vi "Channels.Inline.Block Data Ref to Descriptor (Single).vi"(8 "error in (no error)":errorcluster, 11 "Block Data Ref":T3 {"Data Reference" format="%.0x"}) -> (0 "error out":errorcluster, 3 "Channel Block Descriptor":T1)   [LabVIEW 2016, in "VeriStand Data.lvlib"]
uses:
  VeriStand Data.lvlib
  <vilib>/NI Veristand/Custom Device API/Block Data Reference.ctl
  <vilib>/NI Veristand/Custom Device API/Data Reference.ctl
  Typedefs/Typedefs.Block Descriptor.Channel Block.ctl
  Typedefs/Typedefs.Block Descriptor.ctl
  Channels.Inline.Reference Error Handler.vi
  <vilib>/NI Veristand/Custom Device API/Global Data Refs.vi
  <vilib>/NI Veristand/Custom Device API/Custom Device API.lvlib
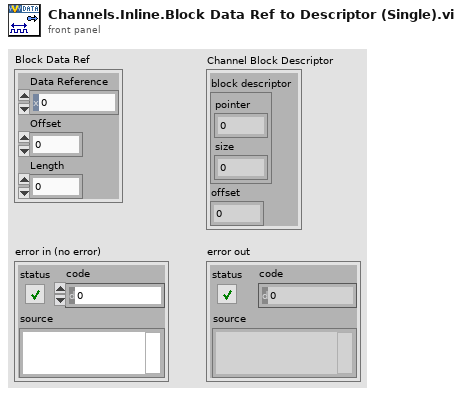
[diagram p1: front panel]
types:
  T1 = typedef "VeriStand Data.lvlib/Typedefs.Block Descriptor.Channel Block.ctl" = cluster{"block descriptor":T2, "offset":u64}
  T2 = typedef "VeriStand Data.lvlib/Typedefs.Block Descriptor.ctl" = cluster{"pointer":u64, "size":u64}
  T3 = typedef "Custom Device API.lvlib/Block Data Reference.ctl" = cluster{"Data Reference":T4, "Offset":u64, "Length":u64}
  T4 = typedef "Custom Device API.lvlib/Data Reference.ctl" = i32
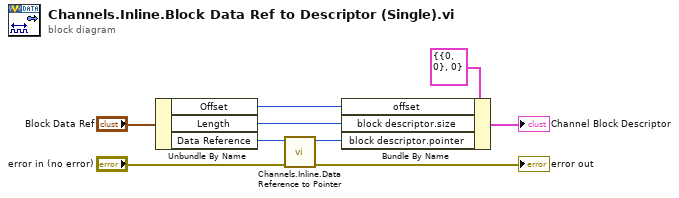
[diagram p0: block diagram]
diagram:
  n1 = Unbundle By Name("Block Data Ref") -> ("Offset"=w3:u64, "Length"=w6:u64, "Data Reference"=w9:T4)
  n2 = call "Channels.Inline.Data Reference to Pointer.vi"("error in (no error)"="error in (no error)", "Data Reference in"=w9) -> ("error out"=→"error out":errorcluster, "Channel Pointer"=w7:u64)  [unwired: 8 in]
  n3 = Bundle By Name(cluster=T1 {"block descriptor"={"pointer"=0, "size"=0}, "offset"=0} ("double block"), "offset"=w3, "block descriptor.size"=w6, "block descriptor.pointer"=w7) -> (→"Channel Block Descriptor":T1)
